vi "servo_pickup_sequence.vi"(0 "servo 3":u8=45) -> ()   [LabVIEW 2017]
uses:
  GlobalVar.vi
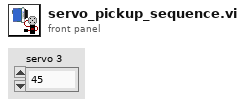
[diagram p1: front panel]
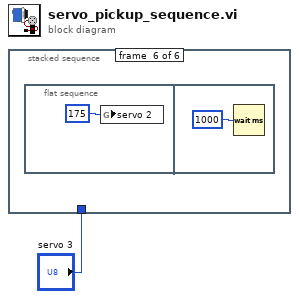
[diagram p0: block diagram]
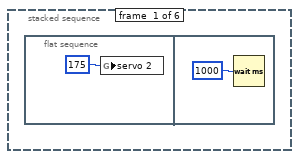
[diagram p2: hidden frame]
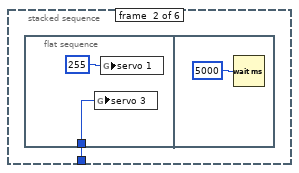
[diagram p3: hidden frame]
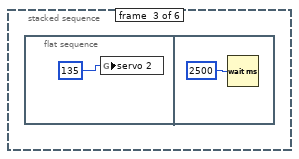
[diagram p4: hidden frame]
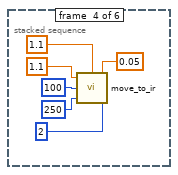
[diagram p5: hidden frame]
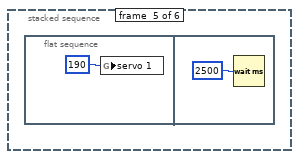
[diagram p6: hidden frame]
diagram:
  n1 = stacked-sequence {
    tunnel: "servo 3" -> [_ w4 _ _ _ _]
    frame #0 {
      n2 = flat-sequence {
        frame #0 {
          n3 = global write "GlobalVar.vi" "servo 2"(u8 175 ("servo 1")) -> ()
        }
        frame #1 {
          n4 = Wait (ms)(milliseconds to wait=u32 1000) -> ()  [unwired: 1 out]
        }
      }
    }
    frame #1 {
      n5 = flat-sequence {
        tunnel: w4 -> [w5]
        frame #0 {
          n6 = global write "GlobalVar.vi" "servo 3"(w5) -> ()
          n7 = global write "GlobalVar.vi" "servo 1"(u8 255 ("servo 1")) -> ()
        }
        frame #1 {
          n8 = Wait (ms)(milliseconds to wait=u32 5000) -> ()  [unwired: 1 out]
        }
      }
    }
    frame #2 {
      n9 = flat-sequence {
        frame #0 {
          n10 = global write "GlobalVar.vi" "servo 2"(u8 135 ("servo 1")) -> ()
        }
        frame #1 {
          n11 = Wait (ms)(milliseconds to wait=u32 2500) -> ()  [unwired: 1 out]
        }
      }
    }
    frame #3 {
      n12 = call "move_to_ir.vi"("step"=2, "precision"=0.05, "target_ir_r"=1.1 ("target_ir_l"), "samples"=250, "delay_after"=u32 100, "target_ir_l"=1.1) -> ()
    }
    frame #4 {
      n13 = flat-sequence {
        frame #0 {
          n14 = global write "GlobalVar.vi" "servo 1"(u8 190 ("servo 1")) -> ()
        }
        frame #1 {
          n15 = Wait (ms)(milliseconds to wait=u32 2500) -> ()  [unwired: 1 out]
        }
      }
    }
    frame #5 {
      n16 = flat-sequence {
        frame #0 {
          n17 = global write "GlobalVar.vi" "servo 2"(u8 175 ("servo 1")) -> ()
        }
        frame #1 {
          n18 = Wait (ms)(milliseconds to wait=u32 1000) -> ()  [unwired: 1 out]
        }
      }
    }
  }
